vi "Square Pulse Plot.vi"(8 "Error In":errorcluster, 9 "Center on Midpoint":bool, 10 "Square Pulse Parameters":T1, 11 "t Array":dbl[](array[numeric])) -> (0 "Error Out":errorcluster, 3 "Square Pulse Plot":cluster{dbl[], dbl[]})   [LabVIEW 2021, in "Fits.lvlib"]
uses:
  Square Pulse Parameters.ctl
  Fits.lvlib
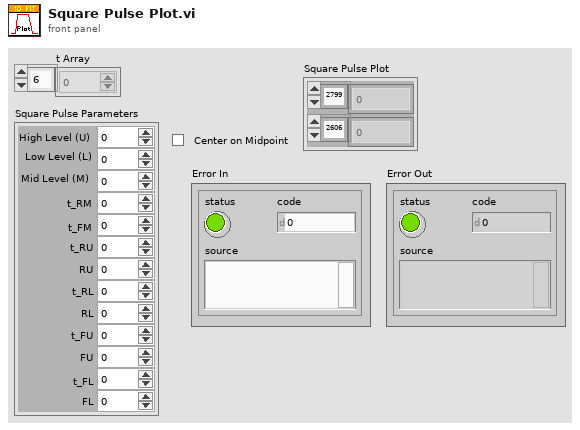
[diagram p1: front panel]
types:
  T1 = typedef "Fits.lvlib/Square Pulse Parameters.ctl" = cluster{"High Level (U)":dbl, "Low Level (L)":dbl, "Mid Level (M)":dbl, "t_RM":dbl, "t_FM":dbl, "t_RU":dbl, "RU":dbl, "t_RL":dbl, "RL":dbl, "t_FU":dbl, "FU":dbl, "t_FL":dbl, "FL":dbl}
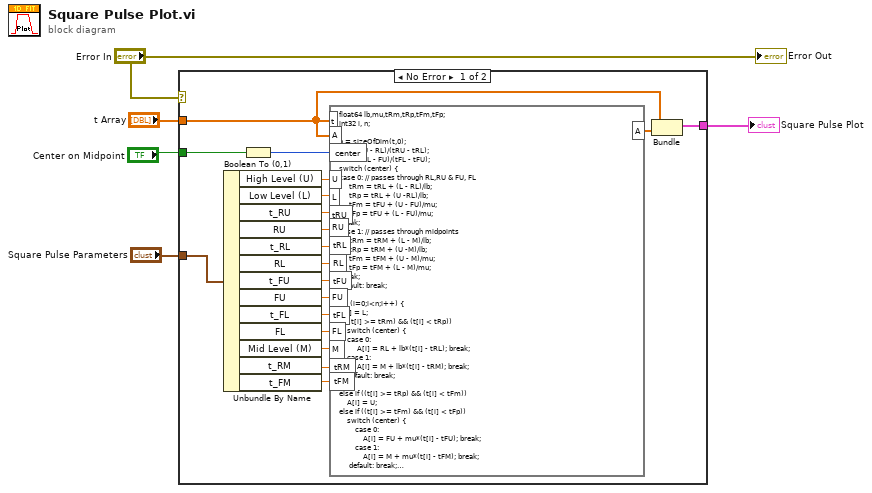
[diagram p0: block diagram]
diagram:
  n1 = case shown="No Error" "Error In" {
    tunnel: "Square Pulse Parameters" -> [w24 _]
    tunnel: "t Array" -> [w11 _]
    tunnel: [w12 _] -> w3
    tunnel: "Center on Midpoint" -> [w10 _]
    frame No Error {
      n2 = Unbundle By Name(w24) -> ("High Level (U)"=w23:dbl, "Low Level (L)"=w22:dbl, "t_RU"=w21:dbl, "RU"=w20:dbl, "t_RL"=w19:dbl, "RL"=w18:dbl, "t_FU"=w17:dbl, "FU"=w16:dbl, "t_FL"=w15:dbl, "FL"=w14:dbl, "Mid Level (M)"=w8:dbl, "t_RM"=w7:dbl, "t_FM"=w6:dbl)
      n3 = Boolean To (0,1)(Boolean=w10) -> (0, 1=w9:i16)
      n4 = formula code="float64 lb,mu,tRm,tRp,tFm,tFp;\nint32 i, n;\n\nn = sizeOfDim(t,0);\nlb = (RU - RL)/(tRU - tRL);\nmu = (FL - FU)/(tFL - tFU);\nswitch (center) {\ncase 0: // passes through RL,RU & FU, FL\n     tRm = tRL + (L - RL)/lb;\n     tRp = tRL + (U -RL)/lb;\n     tFm = tFU + (U - FU)/mu;\n     tFp = tFU + (L - FU)/mu;\nbreak;\ncase 1: // passes through midpoints\n     tRm = tRM + (L - M)/lb;\n     tRp = tRM + (U -M)/lb;\n     tFm = tFM + (U - M)/mu;\n     tFp = tFM + (L - M)/mu;\nbreak;\ndefault: break;\n}\nfor (i=0;i<n;i++) {\nA[i] = L;\nif ((t[i] >= tRm) && (t[i] < tRp))\n    switch (center) {\n    case 0:\n         A[i] = RL + lb*(t[i] - tRL); break;\n    case 1:\n         A[i] = M + lb*(t[i] - tRM); break;\n    default: break;\n    }\nelse if ((t[i] >= tRp) && (t[i] < tFm))\n    A[i] = U;\nelse if ((t[i] >= tFm) && (t[i] < tFp))\n    switch (center) {\n        case 0:\n            A[i] = FU + mu*(t[i] - tFU); break;\n        case 1:\n            A[i] = M + mu*(t[i] - tFM); break;\n     default: break;\n    }\nelse\n    A[i] = L;\n}"("t"=w11, "U"=w23, "L"=w22, "tRU"=w21, "RU"=w20, "tRL"=w19, "RL"=w18, "tFU"=w17, "FU"=w16, "tFL"=w15, "FL"=w14, "A"=w11, "center"=w9, "M"=w8, "tRM"=w7, "tFM"=w6) -> ("A"=w13:dbl[])
      n5 = Bundle("t Array"=w11, "A"=w13) -> (w12:cluster{"t Array":dbl[], "A":dbl[]})  [unwired: 1 in]
    }
    frame Error {
    }
  }
  "Square Pulse Plot" <- w3
  "Error Out" <- "Error In"
